vi "Subset Data by Frequency.vi"(5 "Test Type":string, 7 "Stop Frequency":dbl, 9 "Channel Data":dbl[](array[numeric]), 10 "Frequency Data":dbl[](array[numeric]), 11 "Start Frequency":dbl) -> (1 "Channel Data 2":dbl[](array[numeric]), 2 "Frequency Data 2":dbl[](array[numeric]))   [LabVIEW 2011]
panel:
  out "Length":i32
  out "0 Index":i32
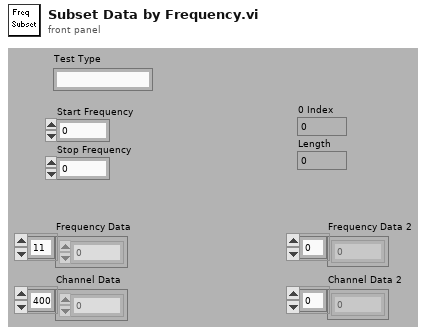
[diagram p1: front panel]
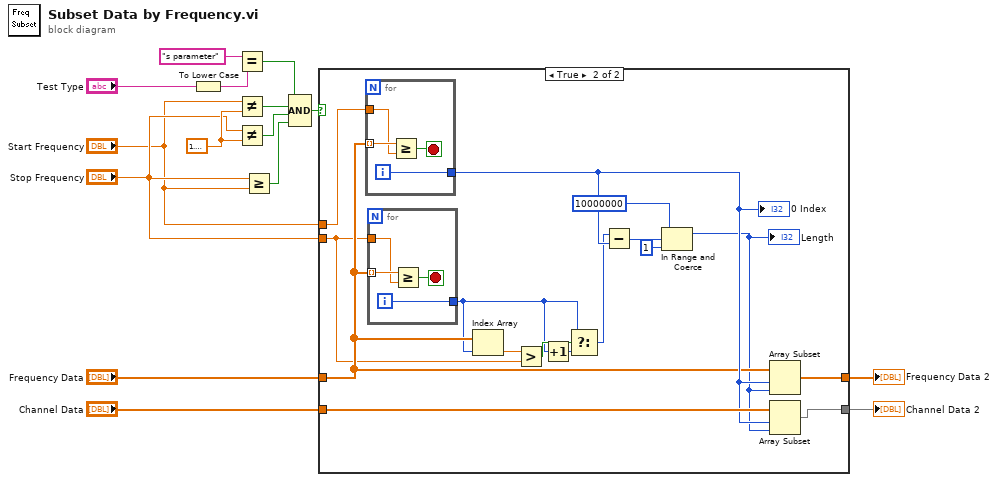
[diagram p0: block diagram]
diagram:
  w6 = 1.1447298858494002
  n1 = To Lower Case(string="Test Type") -> (all lower case string=w14:string)
  n2 = Equal?(x="s parameter", y=w14) -> (x = y?=w13:bool)
  n3 = Not Equal?(x="Start Frequency", y=w6) -> (x != y?=w12:bool)
  n4 = Not Equal?(x="Stop Frequency", y=w6) -> (x != y?=w11:bool)
  n5 = Greater Or Equal?(x="Stop Frequency", y="Start Frequency") -> (x >= y?=w5:bool)
  n6 = Compound Arithmetic op=AND(w13, w12, w11, w5) -> (w10:bool)
  n7 = case shown="True" w10 {
    tunnel: "Frequency Data" -> [w17 w27]
    tunnel: [w17 w30] -> w9
    tunnel: "Channel Data" -> [w16 w32]
    tunnel: [w16 w29] -> w7
    tunnel: "Start Frequency" -> [_ w33]
    tunnel: "Stop Frequency" -> [_ w25]
    frame False {
    }
    frame True {
      n8 = for {
        tunnel: w27 -> [w39] mode=indexing
        tunnel: w33 -> [w38]
        tunnel: [w40] -> w31
        i -> [w40]
        stop <- w41 stop-if-true
        n9 = Greater Or Equal?(x=w39, y=w38) -> (x >= y?=w41:bool)
      }
      "0 Index" <- w31
      n10 = for {
        tunnel: w27 -> [w35] mode=indexing
        tunnel: w25 -> [w34]
        tunnel: [w36] -> w23
        i -> [w36]
        stop <- w37 stop-if-true
        n11 = Greater Or Equal?(x=w35, y=w34) -> (x >= y?=w37:bool)
      }
      n12 = Index Array(array=w27, index=w23) -> (element=w26:dbl)
      n13 = Greater?(x=w26, y=w25) -> (0:w24:bool)
      n14 = Increment(x=w23) -> (x+1=w22:i32)
      n15 = Select(t=w23, s=w24, f=w22) -> (s? t:f=w28:i32)
      n16 = Subtract(x=w28, y=w31) -> (x-y=w21:i32)
      n17 = In Range and Coerce(upper limit=10000000 ("lower limit"), x=w21, lower limit=1) -> (coerced(x)=w18:i32)  [unwired: 1 out]
      "Length" <- w18
      n18 = Array Subset(array=w27, index=w31, length=w18) -> (w30:dbl[])
      n19 = Array Subset(array=w32, index=w31, length=w18) -> (w29:dbl[])
    }
  }
  "Frequency Data 2" <- w9
  "Channel Data 2" <- w7
